vi "Close.vi"(8 "Error In":errorcluster, 11 "Panel In":refnum<class "Panel.lvclass">) -> (0 "Error Out":errorcluster)   [LabVIEW 2023, in "Panel Actor.lvlib" / "Panel.lvlib" / "Panel.lvclass"]
doc: "Closes the Panel.\n\n<B>Panel In:</B> Panel object to close\n<B>Error In:</B> Describes error conditions that occur before this node runs.\n\n<B>Error Out:</B> Contains error information.\n----\nPlease see the following web address for additional documentation and tutorial information:\nhttp://www.mooregoodideas.com/mgi-panel-manager/\n\nAuthor: Derek Trepanier\n\nCopyright (c) 2018, Moore Good Ideas, Inc.\n\nAll rights reserved.\n\nRedistribution and use in source and binary forms, with or without modification, are permitted provided that the following conditions are met:\n\n * Redistributions of source code must retain the above copyright notice, this list of conditions and the following disclaimer.\n * Redistributions in binary form must reproduce the above copyright notice, this list of conditions and the following disclaimer in the documentation and/or other materials provided with the distribution.\n * Neither the name of Moore Good Ideas, Inc. nor the names of its contributors may be used to endorse or promote products derived from this software without specific prior written permission.\n\nTHIS SOFTWARE IS PROVIDED BY THE COPYRIGHT HOLDERS AND CONTRIBUTORS \"AS IS\" AND ANY EXPRESS OR IMPLIED WARRANTIES, INCLUDING, BUT NOT LIMITED TO, THE IMPLIED WARRANTIES OF MERCHANTABILITY AND FITNESS FOR A PARTICULAR PURPOSE ARE DISCLAIMED. IN NO EVENT SHALL THE COPYRIGHT OWNER OR CONTRIBUTORS BE LIABLE FOR ANY DIRECT, INDIRECT, INCIDENTAL, SPECIAL, EXEMPLARY, OR CONSEQUENTIAL DAMAGES (INCLUDING, BUT NOT LIMITED TO, PROCUREMENT OF SUBSTITUTE GOODS OR SERVICES; LOSS OF USE, DATA, OR PROFITS; OR BUSINESS INTERRUPTION) HOWEVER CAUSED AND ON ANY THEORY OF LIABILITY, WHETHER IN CONTRACT, STRICT LIABILITY, OR TORT (INCLUDING NEGLIGENCE OR OTHERWISE) ARISING IN ANY WAY OUT OF THE USE OF THIS SOFTWARE, EVEN IF ADVISED OF THE POSSIBILITY OF SUCH DAMAGE."
uses:
  Panel.lvclass
  Panel.lvclass/Panel.ctl
  Panel Helper/Panel Helper.lvclass
  Panel Registry/Panel Registry.lvclass
  Panel.lvlib
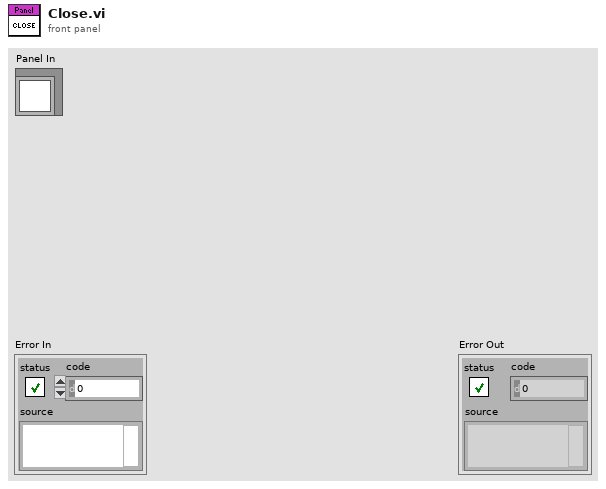
[diagram p1: front panel]
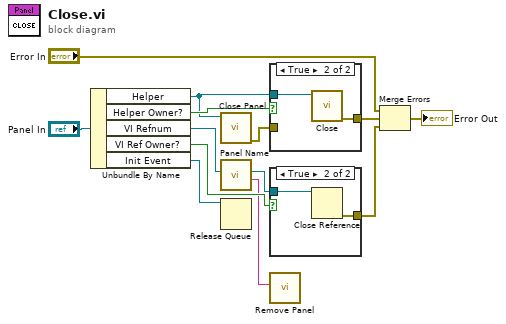
[diagram p0: block diagram]
diagram:
  n1 = Unbundle By Name("Panel In") -> ("Helper"=w6:refnum<class "Panel Helper.lvclass">, "Helper Owner?"=w11:bool, "VI Refnum"=w4:refnum<vi>, "VI Ref Owner?"=w9:bool, "Init Event"=w1:refnum<queue>)
  n2 = call "Close Panel.vi"("Panel Helper in"=w6) -> ("error out"=w5:errorcluster)  [unwired: 10 in]
  n3 = call "Panel Name.vi"("VI in"=w4) -> ("Name"=w2:string, "VI out"=w3:refnum<vi>)  [unwired: 9 in]
  n4 = Release Queue(queue=w1) -> ()  [unwired: 2 in, 3 out]
  n5 = case shown="True" w11 {
    tunnel: w6 -> [_ w15]
    tunnel: [_ w14] -> w10
    tunnel: w5 -> [_ _]
    frame False {
    }
    frame True {
      n6 = call "Close.vi"("Controller in"=w15) -> ("error out"=w14:errorcluster)  [unwired: 10 in]
    }
  }
  n7 = case shown="True" w9 {
    tunnel: [_ w17] -> w8
    tunnel: w3 -> [_ w16]
    frame False {
    }
    frame True {
      n8 = Close Reference(reference=w16) -> (error out=w17:errorcluster)  [unwired: 1 in]
    }
  }
  n9 = call "Remove Panel.vi"("Panel"=w2) -> ()  [unwired: 10 in, 1 out]
  n10 = Merge Errors("Error In", w10, w8) -> (→"Error Out":errorcluster)
